vi "Create G-CLI Script VIPInstall.vi"(8 "error in (no error)":errorcluster, 10 "VIP File Path":path, 11 "PostBuildSupport in":refnum<class "PostBuildSupport.lvclass">) -> (0 "error out":errorcluster, 2 "command":string, 3 "PostBuildSupport out":refnum<class "PostBuildSupport.lvclass">)   [LabVIEW 2019, in "PostBuildSupport.lvclass"]
uses:
  PostBuildSupport.lvclass
  PostBuildSupport.lvclass/PostBuildSupport.ctl
  VIPM/VIPM.lvlib
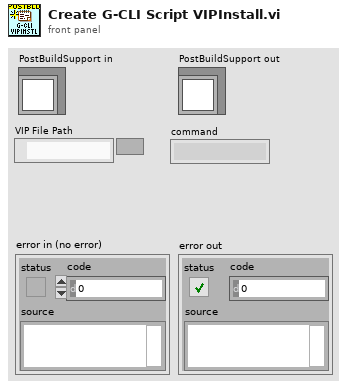
[diagram p1: front panel]
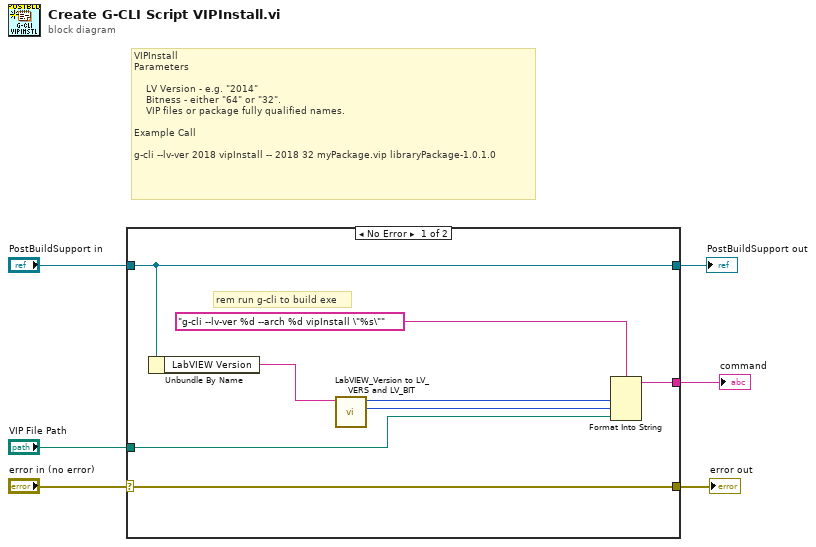
[diagram p0: block diagram]
diagram:
  # "VIPInstall\nParameters\n\n    LV Version - e.g. \"2014\"\n    Bitness - either \"64\" or \"32\".\n    VIP files or package fully qualified names.\n\nExample Call\n\ng-cli --lv-ver 2018 vipInstall -- 2018 32 myPackage.vip libraryPackage-1.0.1.0"
  n1 = case shown="No Error" "error in (no error)" {
    selector: "error in (no error)" -> [w11 w16]
    tunnel: "PostBuildSupport in" -> [w14 w15]
    tunnel: [w11 w16] -> w4
    tunnel: [w14 w15] -> w3
    tunnel: [w12 _] -> w2
    tunnel: "VIP File Path" -> [w10 _]
    frame No Error {
      # "rem run g-cli to build exe"
      n2 = Unbundle By Name(w14) -> ("LabVIEW Version"=w9:string)
      n3 = call "LabVIEW_Version to LV_VERS and LV_BIT.vi"("Package_LabVIEW_Version"=w9) -> ("LV_BIT"=w8:u32, "LV_VER"=w7:u32)  [unwired: 9 in]
      n4 = Format Into String(format string="g-cli --lv-ver %d --arch %d vipInstall \"%s\"", w7, w8, w10) -> (resulting string=w12:string)  [unwired: 2 in, 1 out]
    }
    frame Error {
    }
  }
  "error out" <- w4
  "PostBuildSupport out" <- w3
  "command" <- w2
